vi "EditLimsTestStepValues.vi"(8 "error in (no error)":errorcluster, 11 "ByteGSAPIBase in":refnum<class "ByteGSAPIBase.lvclass">) -> (0 "error out":errorcluster, 3 "ByteGSAPIBase out":refnum<class "ByteGSAPIBase.lvclass">)   [LabVIEW 2019, in "ByteGSWebAPI.lvlib" / "ByteGSAPIBase.lvclass"]
uses:
  ByteGSAPIBase.lvclass
  TypeDef/UpdateLimsTestStepData.ctl
  ByteGSAPIBase.lvclass/ByteGSAPIBase.ctl
  <vilib>/Bytelabs/ByteREST/ByteRESTClass/ByteRESTBase/RESTBase.lvclass
panel:
  out "step result":T1
  in  "step-id":u32
  in  "value":dbl
  in  "duration hours":dbl
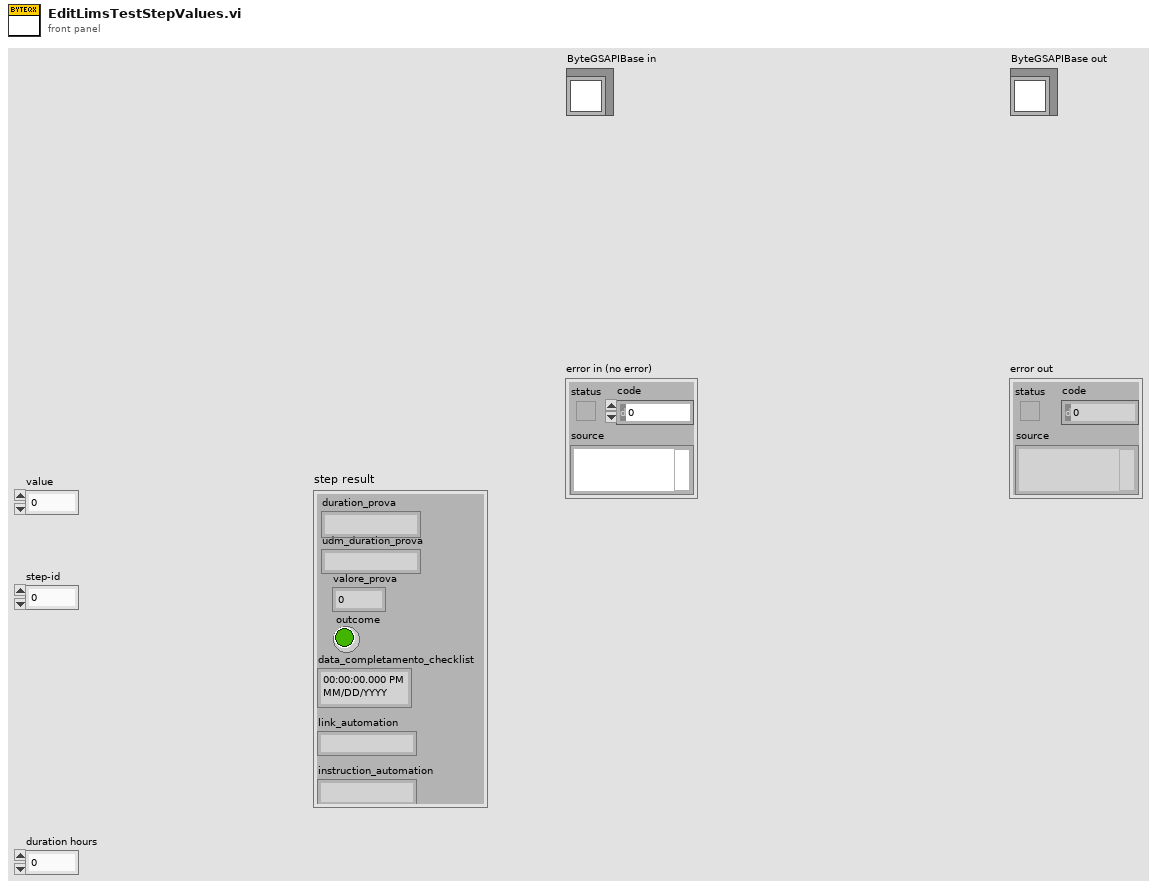
[diagram p1: front panel]
types:
  T1 = typedef "ByteGSWebAPI.lvlib/ByteGSAPIBase.lvclass/UpdateLimsTestStepData.ctl" = cluster{"outcome":bool, "data_completamento_checklist":timestamp, "udm_duration_prova":string, "valore_prova":dbl, "link_automation":string, "instruction_automation":string, "duration_prova":string}
  T2 = cluster{"duration_prova":string, "udm_duration_prova":string, "data_completamento_checklist":string, "valore_prova":dbl, "outcome":string, "link_automation":string, "instruction_automation":string}
  T3 = typedef "ByteGSWebAPI.lvlib/ByteGSAPIBase.lvclass/Step.ctl" = cluster{"id":i32, "descrizione":string, "prova":string, "assets":T4[], "criterio_accettazione":string, "valore_criterio_accettazione_max":dbl, "valore_criterio_accettazione_min":dbl, "udm_criterio_accettazione":string, "duration_prova":string, "udm_duration_prova":string, "valore_prova":dbl, "ordine":i32, "user":i32, "link_automation":string, "instruction_automation":string, "data_completamento_checklist":timestamp, "outcome":bool}
  T4 = typedef "ByteGSWebAPI.lvlib/ByteGSAPIBase.lvclass/Asset.ctl" = cluster{"descrizione":string, "slug":string, "id":i32}
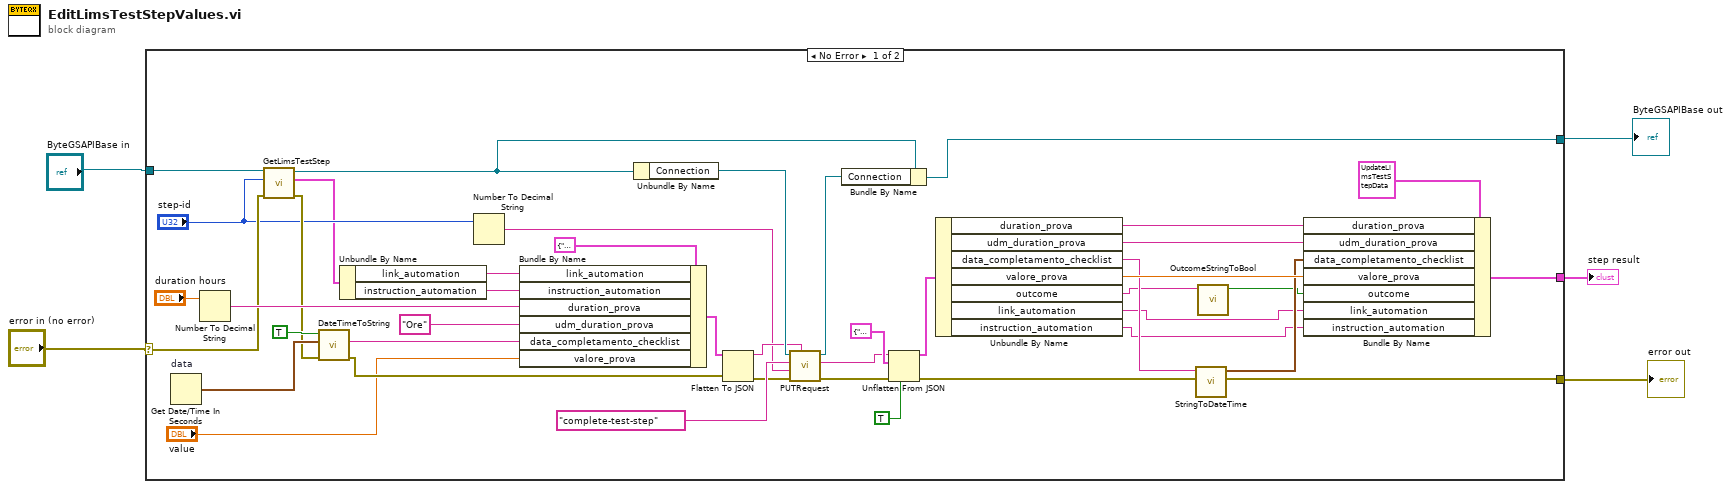
[diagram p0: block diagram]
diagram:
  n1 = case shown="No Error" "error in (no error)" {
    selector: "error in (no error)" -> [w17 w50]
    tunnel: [w25 w50] -> w4
    tunnel: [w47 w49] -> w3
    tunnel: "ByteGSAPIBase in" -> [w6 w49]
    tunnel: [w26 _] -> w5
    frame No Error {
      n2 = Get Date/Time In Seconds "data"() -> (seconds since 1Jan1904=w20:timestamp)
      n3 = Number To Decimal String(number="duration hours") -> (decimal integer string=w41:string)  [unwired: 1 in]
      n4 = call-dynamic "GetLimsTestStep.vi"("error in (no error)"=w17, "step-id"="step-id", "ByteGSAPIBase in"=w6) -> ("error out"=w16:errorcluster, "StepList"=w14:T3, "ByteGSAPIBase out"=w18:refnum<class "ByteGSAPIBase.lvclass">)  [unwired: 6 in]
      n5 = call "DateTimeToString.vi"("error in"=w16, "current time"=w20, "include Time?"=TRUE ("Time")) -> ("error out"=w38:errorcluster, "date string"=w39:string)  [unwired: 7 in]
      n6 = Unbundle By Name(w14) -> ("link_automation"=w13:string, "instruction_automation"=w12:string)
      n7 = Number To Decimal String(number="step-id") -> (decimal integer string=w23:string)  [unwired: 1 in]
      n8 = Bundle By Name(cluster=T2 {"duration_prova"="3", "udm_duration_prova"="Ore", "data_completamento_checklist"="2024-10-24T17:19:12Z", "valore_prova"=5.0, "outcome"="P", "link_automation"="", "instruction_automation"=""} ("Update Step"), "link_automation"=w13, "instruction_automation"=w12, "duration_prova"=w41, "udm_duration_prova"="Ore", "data_completamento_checklist"=w39, "valore_prova"="value") -> (w40:T2)
      n9 = Unbundle By Name(w18) -> ("Connection"=w48:refnum<class "RESTBase.lvclass">)
      n10 = Flatten To JSON(anything=w40, error in (no error)=w38) -> (JSON string=w44:string, 11:w43:errorcluster)  [unwired: 1 in]
      n11 = call-dynamic "PUTRequest.vi"("Body in"=w44, "error in (no error)"=w43, "Parameter"=w23, "Request"="complete-test-step", "ByteRESTBase in"=w48) -> ("error out"=w28:errorcluster, "Body"=w27:string, "ByteRESTBase out"=w46:refnum<class "RESTBase.lvclass">)  [unwired: 3 in, 1 out]
      n12 = Bundle By Name(cluster=w18, "Connection"=w46) -> (w47:refnum<class "ByteGSAPIBase.lvclass">)
      n13 = Unflatten From JSON(JSON string=w27, type and defaults=T2 {"duration_prova"="", "udm_duration_prova"="", "data_completamento_checklist"="", "valore_prova"=0.0, "outcome"="P", "link_automation"="", "instruction_automation"=""}, default null elements? (F)=TRUE, error in (no error)=w28) -> (value=w35:T2, error out=w29:errorcluster)  [unwired: 3 in]
      n14 = Unbundle By Name(w35) -> ("duration_prova"=w34:string, "udm_duration_prova"=w33:string, "data_completamento_checklist"=w31:string, "valore_prova"=w32:dbl, "outcome"=w8:string, "link_automation"=w9:string, "instruction_automation"=w10:string)
      n15 = call "StringToDateTime.vi"("error in (no error)"=w29, "datetime string"=w31) -> ("error out"=w25:errorcluster, "timestamp"=w30:timestamp)  [unwired: 8 in]
      n16 = call "OutcomeStringToBool.vi"("outcome string"=w8) -> ("outcome bool"=w7:bool)  [unwired: 10 in]
      n17 = Bundle By Name(cluster=T1 {"outcome"=FALSE, "data_completamento_checklist"=timestamp(0 s since 1904-01-01), "udm_duration_prova"="", "valore_prova"=0.0, "link_automation"="", "instruction_automation"="", "duration_prova"=""} ("Result Step"), "duration_prova"=w34, "udm_duration_prova"=w33, "data_completamento_checklist"=w30, "valore_prova"=w32, "outcome"=w7, "link_automation"=w9, "instruction_automation"=w10) -> (w26:T1)
    }
    frame Error {
    }
  }
  "error out" <- w4
  "ByteGSAPIBase out" <- w3
  "step result" <- w5
